vi "XY Plot - Y Scale - Marker Position Left--Const.vi"() -> (3 "Y Scale.Marker.Position:Left":i32)   [LabVIEW 2017, in "DTacq Plot Display Library.lvlib"]
uses:
  DTacq Plot Display Library.lvlib
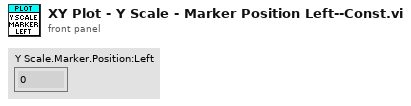
[diagram p1: front panel]
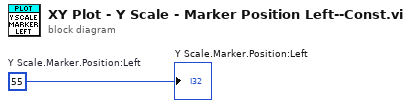
[diagram p0: block diagram]
diagram:
  w1 = 55  # Y Scale.Marker.Position:Left
  "Y Scale.Marker.Position:Left" <- w1
